vi "启动界面.vi"() -> ()   [LabVIEW 2018]
panel:
  out "?":string
  out "图片/视频路径":string
  out "图片/视频完整路径":path
  out "模式选择output":i8
  out "是否使用GPU计算output":i8
  out "视频检测帧间隔output":i8
  in  "退出程序-":bool
  in  "模式选择-":bool
  in  "信息说明-":bool
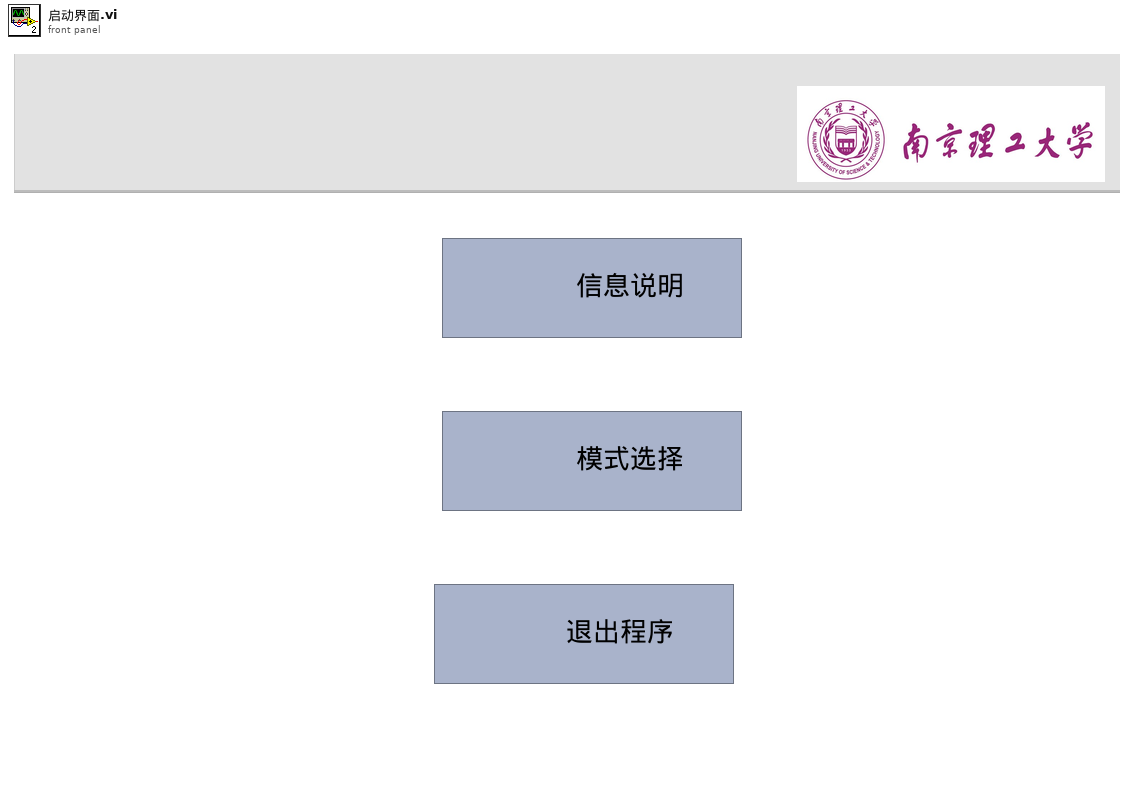
[diagram p1: front panel]
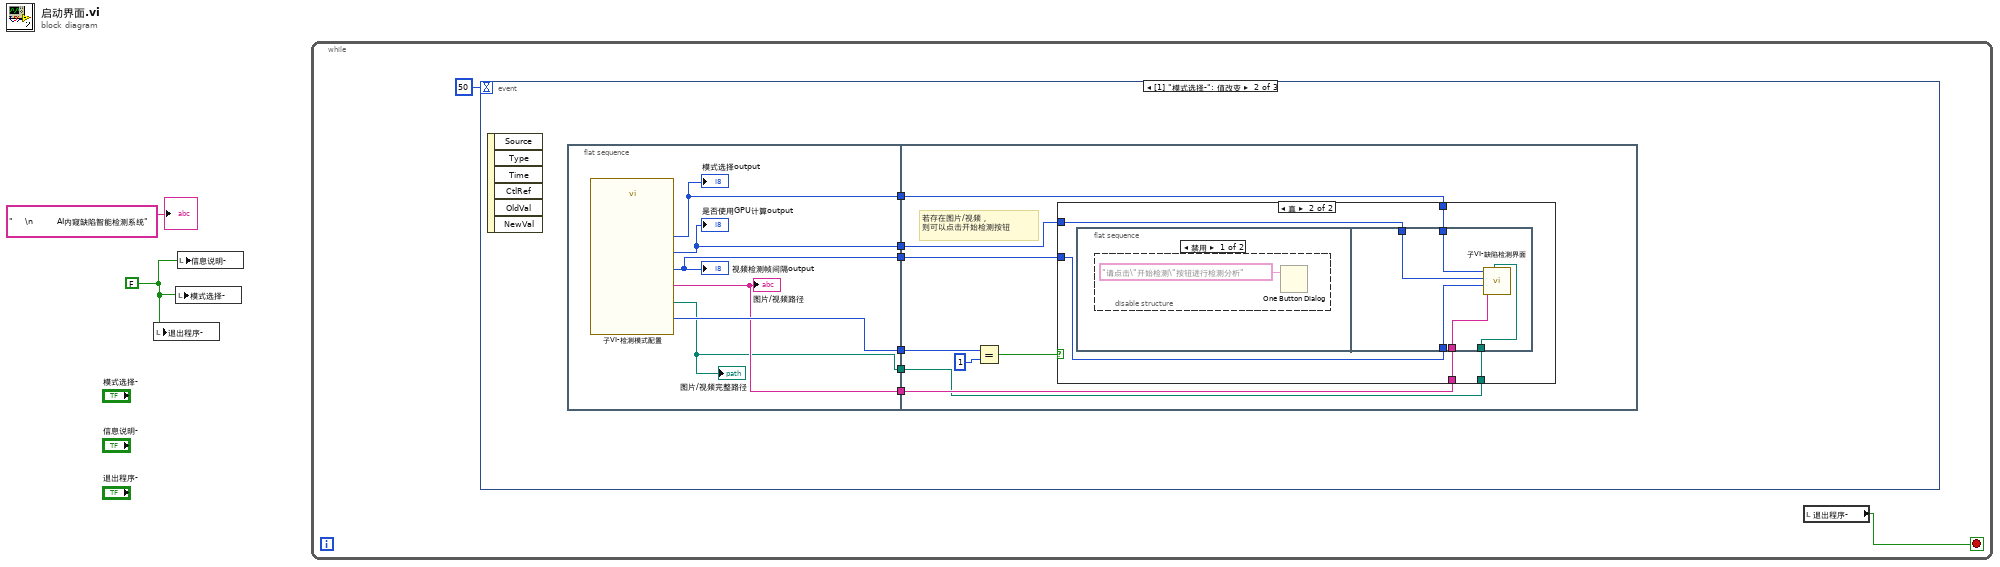
[diagram p0: block diagram]
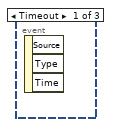
[diagram p2: hidden frame]
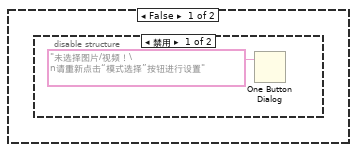
[diagram p3: hidden frame]
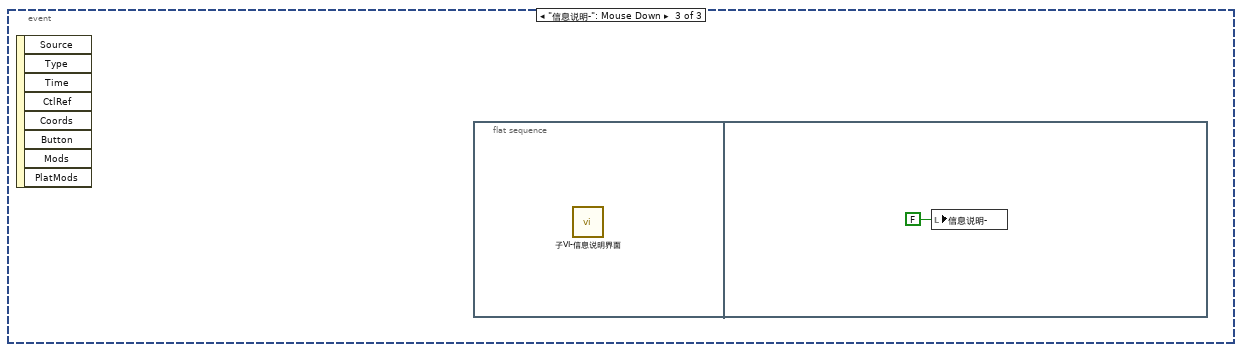
[diagram p6: hidden frame]
diagram:
  w1 = FALSE ("退出程序")
  n1 = local write "退出程序-"(w1) -> ()
  n2 = local write "模式选择-"(w1) -> ()
  n3 = local write "信息说明-"(w1) -> ()
  n4 = while {
    stop <- w4 stop-if-true
    n5 = event shown="[1] \"模式选择-\": 值改变" {
      selector: _ -> [_ _ _]
      dyn-events: _ -> [_ _ _]
      timeout: 50 -> [_ _ _]
      event Timeout {
        n6 = event-data() -> ()  [unwired: 1 in, 3 out]
      }
      event "模式选择-": Value Change {
        n7 = event-data() -> ()  [unwired: 1 in, 6 out]
        n8 = flat-sequence {
          tunnel: [w16] -> w10
          tunnel: [w15] -> w9
          tunnel: [w14] -> w8
          tunnel: [w13] -> w7
          tunnel: [w12] -> w6
          tunnel: [w11] -> w5
          tunnel: w10 -> [w23]
          tunnel: w9 -> [w21]
          tunnel: w8 -> [w20]
          tunnel: w7 -> [w19]
          tunnel: w6 -> [w18]
          tunnel: w5 -> [w17]
          frame #0 {
            n9 = call "子VI-检测模式配置.vi"() -> ("视频检测帧间隔output"=w13:i8, "模式选择output"=w15:i8, "是否使用GPU计算output"=w14:i8, "图片/视频路径"=w12:string, "flag"=w16:i32, "图片/视频完整路径"=w11:path)  [unwired: 4 in]
            "图片/视频路径" <- w12
            "图片/视频完整路径" <- w11
            "模式选择output" <- w15
            "是否使用GPU计算output" <- w14
            "视频检测帧间隔output" <- w13
          }
          frame #1 {
            # "若存在图片/视频，\n则可以点击开始检测按钮"
            n10 = Equal?(x=w23, y=i8 1) -> (x = y?=w22:bool)
            n11 = case shown="真" w22 {
              tunnel: w21 -> [_ w30]
              tunnel: w20 -> [_ w29]
              tunnel: w19 -> [_ w28]
              tunnel: w18 -> [_ w27]
              tunnel: w17 -> [_ w26]
              frame False {
                n12 = disable-structure shown="禁用" {
                  frame Disabled {
                    n13 = One Button Dialog(message="未选择图片/视频！\n请重新点击“模式选择”按钮进行设置" ("消息")) -> ()  [unwired: 1 in, 1 out]
                  }
                  frame Enabled {
                  }
                }
              }
              frame True {
                n14 = flat-sequence {
                  tunnel: w30 -> [w36]
                  tunnel: w29 -> [w35]
                  tunnel: w28 -> [w34]
                  tunnel: w27 -> [w33]
                  tunnel: w26 -> [w32]
                  frame #0 {
                    n15 = disable-structure shown="禁用" {
                      frame Disabled {
                        n16 = One Button Dialog(message="请点击\"开始检测\"按钮进行检测分析" ("消息")) -> ()  [unwired: 1 in, 1 out]
                      }
                      frame Enabled {
                      }
                    }
                  }
                  frame #1 {
                    n17 = call "子VI-缺陷检测界面.vi"(6:"图片/视频路径"=w32, 7:"图片/视频路径"=w33, "视频检测帧间隔output"=w34, "是否使用GPU计算output"=w35, "模式选择output"=w36) -> ()  [unwired: 6 in]
                  }
                }
              }
            }
          }
        }
      }
      event "信息说明-": Mouse Down {
        n18 = event-data() -> ()  [unwired: 1 in, 8 out]
        n19 = flat-sequence {
          frame #0 {
            n20 = call "子VI-信息说明界面.vi"() -> ()  [unwired: 12 in]
          }
          frame #1 {
            n21 = local write "信息说明-"(FALSE ("信息说明-")) -> ()
          }
        }
      }
    }
    n22 = local read "退出程序-"() -> (w4:bool)
  }
  "?" <- "    \n        AI内窥缺陷智能检测系统"
